vi "Alignment Adjustment.vi"(9 "Right Side of Field?":bool, 10 "Distance":dbl, 11 "BB Angle":dbl) -> (3 "X Setpoint":dbl)   [LabVIEW 2011]
panel:
  in  "y":dbl=-1.0
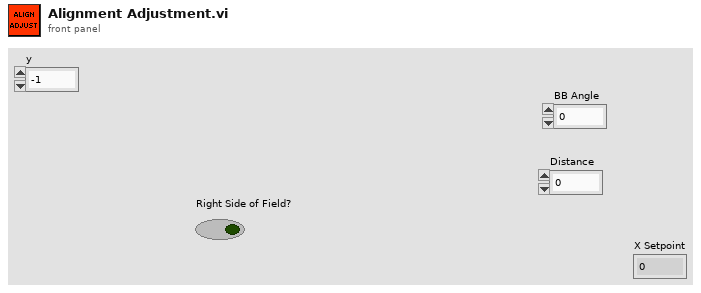
[diagram p1: front panel]
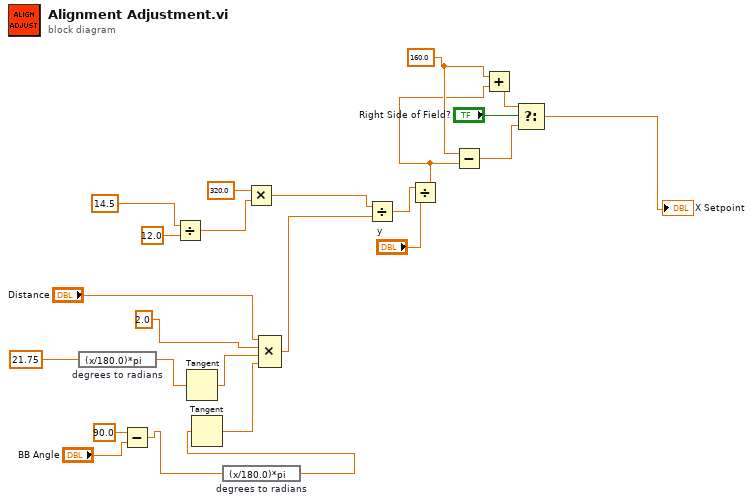
[diagram p0: block diagram]
diagram:
  w9 = 160.0 ("y")
  n1 = expression code="(x/180.0)*pi" "degrees to radians"(21.75 ("x")) -> (w13:dbl)
  n2 = Subtract(x=90.0, y="BB Angle") -> (x-y=w16:dbl)
  n3 = Divide(x=14.5 ("y"), y=12.0) -> (x/y=w10:dbl)
  n4 = Tangent(1:w13) -> (0:w20:dbl)
  n5 = expression code="(x/180.0)*pi" "degrees to radians"(w16) -> (w15:dbl)
  n6 = Tangent(1:w15) -> (0:w21:dbl)
  n7 = Multiply(x=320.0, y=w10) -> (x*y=w5:dbl)
  n8 = Compound Arithmetic op=MULTIPLY("Distance", 2.0 ("y"), w20, w21) -> (w19:dbl)
  n9 = Divide(x=w5, y=w19) -> (x/y=w2:dbl)
  n10 = Divide(x=w2, y="y") -> (x/y=w3:dbl)
  n11 = Subtract(x=w9, y=w3) -> (x-y=w8:dbl)
  n12 = Add(x=w9, y=w3) -> (x+y=w7:dbl)
  n13 = Select(t=w7, s="Right Side of Field?", f=w8) -> (s? t:f=→"X Setpoint":dbl)
